vi "Set UA Folder.vi"(8 "error in (no error)":errorcluster, 9 "Folder Name In":string, 10 "Parent Folder In (opt)":string, 11 "OPC UA server refnum in":T1) -> (0 "error out":errorcluster, 2 "Folder Id Out":string, 3 "OPC UA server refnum out":T1)   [LabVIEW 2024, in "OPCUA.lvlib"]
uses:
  <vilib>/OPCUA/controls/OPC UA Server Refnum.ctl
  OPCUA.lvlib
  <vilib>/OPCUA/NI OPC UA Server.lvlib
panel:
  in  "Description (opt)":string
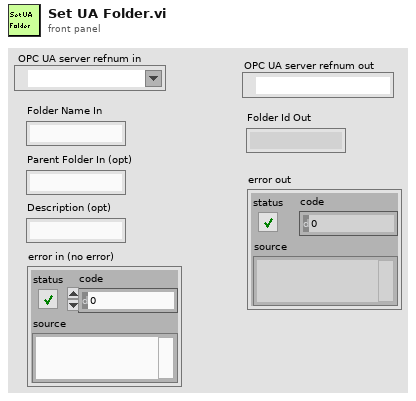
[diagram p1: front panel]
types:
  T1 = typedef "OPC UA Server Refnum.ctl" = refnum<k21>
  T2 = typedef "NodeId.ctl" = string
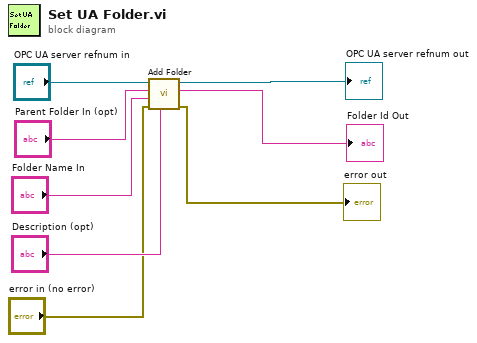
[diagram p0: block diagram]
diagram:
  n1 = call <vilib>:"Add Folder.vi"("description"="Description (opt)", "error in (no error)"="error in (no error)", "folder name"="Folder Name In", "parent folder node ID"="Parent Folder In (opt)", "OPC UA server refnum in"="OPC UA server refnum in") -> ("error out"=→"error out":errorcluster, "folder node ID"=→"Folder Id Out":T2, "OPC UA server refnum out"=→"OPC UA server refnum out":T1)  [unwired: 3 in]
